vi "Valid Library and VI Information Array.vi"(10 "VI Information Array":T1[](array[typedef]), 11 "Engine in":refnum<class "Engine.lvclass">) -> (3 "Valid":bool)   [LabVIEW 2019, in "Engine.lvclass"]
uses:
  Engine.lvclass
  Public/VI Information.ctl
  Engine.lvclass/Engine.ctl
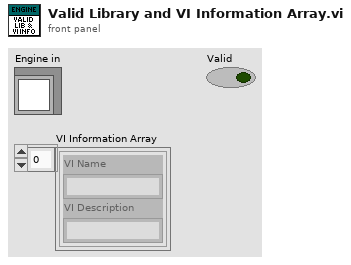
[diagram p1: front panel]
types:
  T1 = typedef "Engine.lvclass/VI Information.ctl" = cluster{"VI Name":string, "VI Description":string}
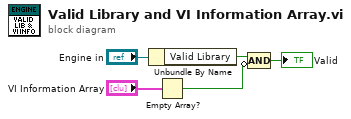
[diagram p0: block diagram]
diagram:
  n1 = Unbundle By Name("Engine in") -> ("Valid Library"=w3:bool)
  n2 = Empty Array?(array="VI Information Array") -> (empty?=w4:bool)
  n3 = Compound Arithmetic op=AND(w3, invert w4) -> (→"Valid":bool)
